vi "YFM2.vi"() -> ()   [LabVIEW 2017]
uses:
  <vilib>/DAQmx/write.llb/DAQmx Write (Analog DBL 1Chan 1Samp).vi
  <vilib>/DAQmx/read.llb/DAQmx Read (Analog Wfm 1Chan NSamp).vi
  <vilib>/DAQmx/create/channels.llb/DAQmx Create Channel (AO-Voltage-Basic).vi
  <vilib>/DAQmx/create/channels.llb/DAQmx Create Channel (AI-Voltage-Basic).vi
  <vilib>/DAQmx/configure/timing.llb/DAQmx Timing (Sample Clock).vi
  <vilib>/DAQmx/miscellaneous.llb/DAQmx Fill In Error Info.vi
  <vilib>/measure/NI_MABase.lvlib
panel:
  out "error out 3":errorcluster={"status"=TRUE, "code"=-200099, "source"="DAQmx Create Channel (AO-Voltage-Basic).vi:1870002<append>\n<B>Task Name: </B>_unnamedTask<0>"}
  in  "error in 3":errorcluster
  out "transfer characteristic":cluster{"Y":dbl[], "Y":dbl[]}(graph)
  in  "Vd":dbl
  in  "Vd channels":tag="Dev3/ao1"
  out "error out 2":errorcluster
  in  "error in 2":errorcluster
  out "error out":errorcluster={"status"=TRUE, "code"=-200477, "source"="YFM.vi<append>\n<B>Task Name: </B>_unnamedTask<1>"}
  in  "Id channels":tag="Dev9/ai0"
  out "# of step":dbl=nan
  in  "Step":dbl=0.1
  in  "Stop (V)":dbl=2.0
  in  "Start (V)":dbl=1.0
  in  "error in":errorcluster
  in  "Vg channels":tag="Dev3/ao0"
  # "Vg"
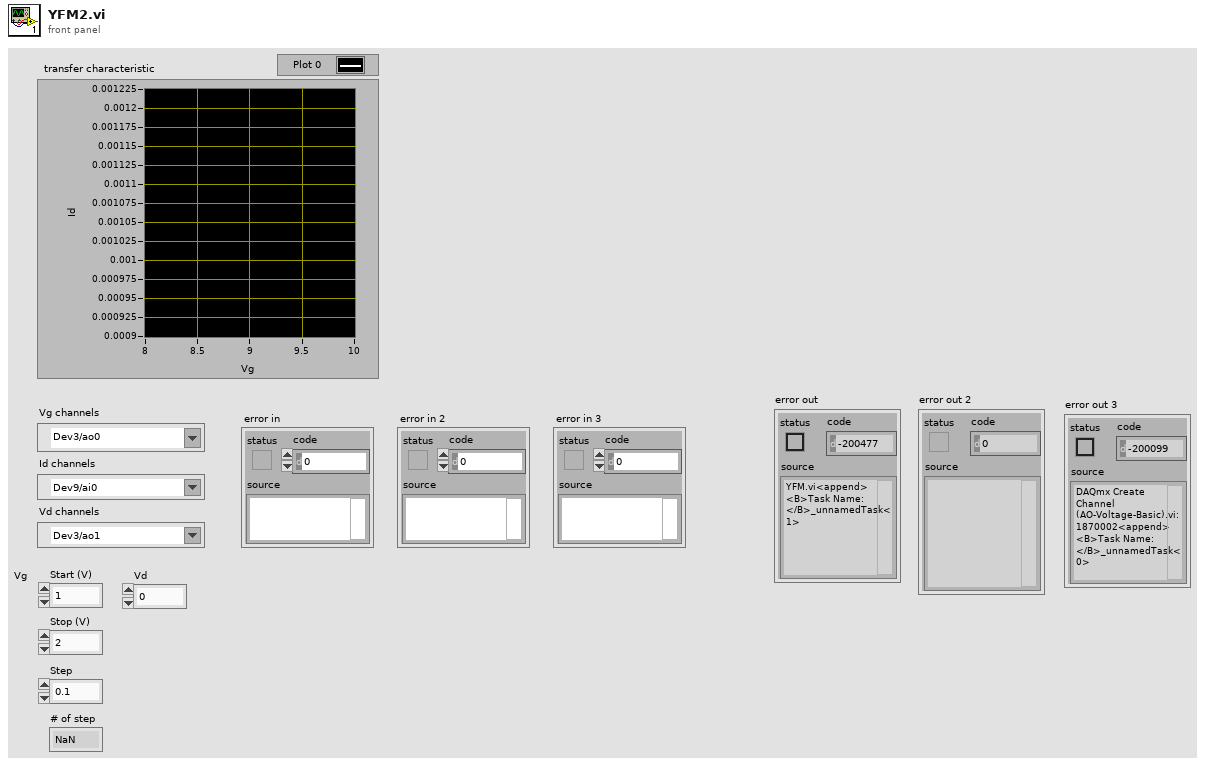
[diagram p1: front panel]
types:
  T1 = cluster{"signal out":waveform(dbl), "data":waveform(dbl)}
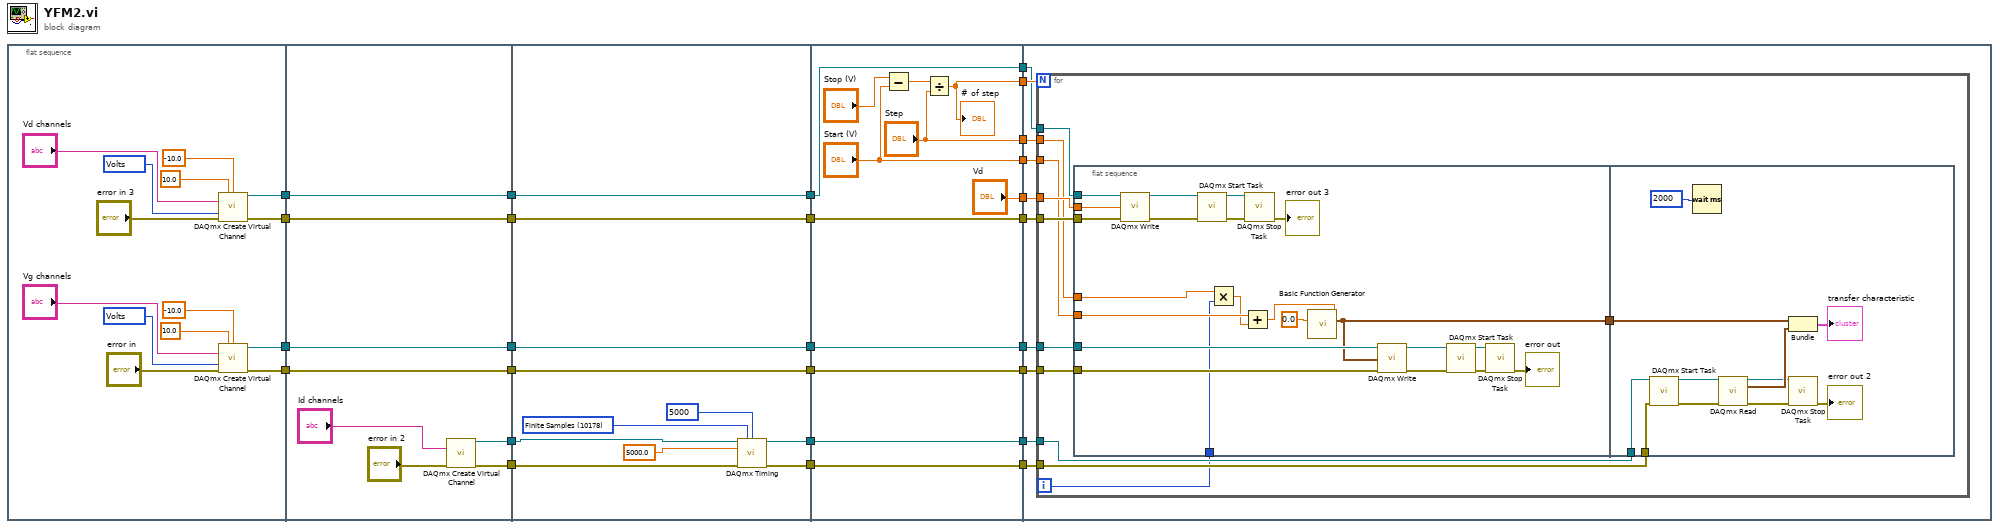
[diagram p0: block diagram]
diagram:
  n1 = flat-sequence {
    tunnel: [w35] -> w15
    tunnel: [w34] -> w13
    tunnel: [w29] -> w5
    tunnel: [w28] -> w1
    tunnel: w15 -> [w48]
    tunnel: [w48] -> w14
    tunnel: w13 -> [w47]
    tunnel: [w47] -> w12
    tunnel: [w44] -> w11
    tunnel: [w43] -> w10
    tunnel: [w42] -> w6
    tunnel: w5 -> [w42]
    tunnel: [w41] -> w2
    tunnel: w1 -> [w41]
    tunnel: w14 -> [w59]
    tunnel: w12 -> [w58]
    tunnel: w11 -> [w57]
    tunnel: w10 -> [w53]
    tunnel: [w59] -> w26
    tunnel: [w58] -> w25
    tunnel: [w52] -> w24
    tunnel: [w51] -> w23
    tunnel: [w50] -> w7
    tunnel: w6 -> [w50]
    tunnel: [w49] -> w3
    tunnel: w2 -> [w49]
    tunnel: w26 -> [w71]
    tunnel: w25 -> [w70]
    tunnel: w24 -> [w69]
    tunnel: w23 -> [w68]
    tunnel: [w71] -> w22
    tunnel: [w70] -> w21
    tunnel: [w69] -> w20
    tunnel: [w68] -> w19
    tunnel: ["Step"] -> w18
    tunnel: ["Start (V)"] -> w17
    tunnel: [w60] -> w16
    tunnel: ["Vd"] -> w9
    tunnel: [w62] -> w8
    tunnel: w7 -> [w62]
    tunnel: [w61] -> w4
    tunnel: w3 -> [w61]
    tunnel: w22 -> [w79]
    tunnel: w21 -> [w78]
    tunnel: w20 -> [w76]
    tunnel: w19 -> [w75]
    tunnel: w18 -> [w81]
    tunnel: w17 -> [w80]
    tunnel: w16 -> [w77]
    tunnel: w9 -> [w74]
    tunnel: w8 -> [w73]
    tunnel: w4 -> [w72]
    frame #0 {
      w31 = 10348 items=["Volts"=10348, "From Custom Scale"=10065] ("units")
      w36 = 10348 items=["Volts"=10348, "From Custom Scale"=10065] ("units")
      n2 = call-poly <vilib>:"DAQmx Create Virtual Channel.vi"("maximum value"=10.0, "minimum value"=-10.0, "physical channels"="Vd channels", "units"=w31, "error in"="error in 3") -> ("task out"=w29:refnum<k21>, "error out"=w28:errorcluster)  [unwired: 9 in]
      n3 = call-poly <vilib>:"DAQmx Create Virtual Channel.vi"("maximum value"=10.0, "minimum value"=-10.0, "physical channels"="Vg channels", "units"=w36, "error in"="error in") -> ("task out"=w35:refnum<k21>, "error out"=w34:errorcluster)  [unwired: 9 in]
    }
    frame #1 {
      n4 = call-poly <vilib>:"DAQmx Create Virtual Channel.vi"("physical channels"="Id channels", "error in"="error in 2") -> ("task out"=w44:refnum<k21>, "error out"=w43:errorcluster)  [unwired: 12 in]
    }
    frame #2 {
      w56 = 10178 items=["Finite Samples"=10178, "Continuous Samples"=10123, "Hardware Timed Single Point"=12522] ("sample mode")
      n5 = call-poly <vilib>:"DAQmx Timing.vi"("task/channels in"=w57, "sample mode"=w56, "samples per channel"=5000, "rate"=5000.0, "error in"=w53) -> ("task out"=w52:refnum<k21>, "error out"=w51:errorcluster)  [unwired: 9 in]
    }
    frame #3 {
      n6 = Subtract(x="Stop (V)", y="Start (V)") -> (x-y=w67:dbl)
      n7 = Divide(x=w67, y="Step") -> (x/y=w60:dbl)
      "# of step" <- w60
    }
    frame #4 {
      n8 = for {
        N: w77 -> [_]
        tunnel: w81 -> [w87]
        tunnel: w80 -> [w86]
        tunnel: w79 -> [w85]
        tunnel: w78 -> [w84]
        tunnel: w76 -> [w92]
        tunnel: w75 -> [w91]
        tunnel: w74 -> [w90]
        tunnel: w73 -> [w89]
        tunnel: w72 -> [w88]
        i -> [w82]
        n9 = flat-sequence {
          tunnel: w90 -> [w114]
          tunnel: w89 -> [w111]
          tunnel: w88 -> [w110]
          tunnel: w87 -> [w106]
          tunnel: w86 -> [w105]
          tunnel: w85 -> [w104]
          tunnel: w84 -> [w103]
          tunnel: [w102] -> w83
          tunnel: w82 -> [w93]
          tunnel: w92 -> [w123]
          tunnel: w91 -> [w122]
          tunnel: w83 -> [w116]
          frame #0 {
            n10 = call-poly <vilib>:"DAQmx Write.vi"("task/channels in"=w111, "data"=w114, "error in"=w110) -> ("task out"=w113:refnum<k21>, "error out"=w109:errorcluster)  [unwired: 10 in, 1 out]
            n11 = call <vilib>:"DAQmx Start Task.vi"("task/channels in"=w113, "error in"=w109) -> ("task out"=w112:refnum<k21>, "error out"=w108:errorcluster)  [unwired: 12 in]
            n12 = Multiply(x=w106, y=w93) -> (x*y=w95:dbl)
            n13 = Add(x=w105, y=w95) -> (x+y=w96:dbl)
            n14 = call <vilib>:"DAQmx Stop Task.vi"("task/channels in"=w112, "error in"=w108) -> ("error out"=→"error out 3":errorcluster)  [unwired: 12 in, 1 out]
            n15 = call <vilib>:"Basic Function Generator.vi"("offset"=w96, "amplitude"=0.0) -> ("signal out"=w102:waveform(dbl))  [unwired: 7 in, 2 out]
            n16 = call-poly <vilib>:"DAQmx Write.vi"("task/channels in"=w104, "data"=w102, "error in"=w103) -> ("task out"=w97:refnum<k21>, "error out"=w98:errorcluster)  [unwired: 10 in, 1 out]
            n17 = call <vilib>:"DAQmx Start Task.vi"("task/channels in"=w97, "error in"=w98) -> ("task out"=w99:refnum<k21>, "error out"=w100:errorcluster)  [unwired: 12 in]
            n18 = call <vilib>:"DAQmx Stop Task.vi"("task/channels in"=w99, "error in"=w100) -> ("error out"=→"error out":errorcluster)  [unwired: 12 in, 1 out]
          }
          frame #1 {
            n19 = call <vilib>:"DAQmx Start Task.vi"("task/channels in"=w123, "error in"=w122) -> ("task out"=w125:refnum<k21>, "error out"=w124:errorcluster)  [unwired: 12 in]
            n20 = Wait (ms)(milliseconds to wait=u32 2000) -> ()  [unwired: 1 out]
            n21 = call-poly <vilib>:"DAQmx Read.vi"("task/channels in"=w125, "error in"=w124) -> ("task out"=w119:refnum<k21>, "data"=w120:waveform(dbl), "error out"=w118:errorcluster)  [unwired: 11 in]
            n22 = Bundle("signal out"=w116, "data"=w120) -> (→"transfer characteristic":T1)  [unwired: 1 in]
            n23 = call <vilib>:"DAQmx Stop Task.vi"("task/channels in"=w119, "error in"=w118) -> ("error out"=→"error out 2":errorcluster)  [unwired: 12 in, 1 out]
          }
        }
      }
    }
  }
